vi "filtering_and_quant_demoinfocom.vi"(9 "Parity Size":dbl, 10 "Quantization rate":dbl) -> (0 "correlation coefficient r":dbl format="%.7g", 1 "SDR1 Key before ECC":u8[](array[numeric]), 2 "SDR2 Key before ECC":u8[](array[numeric]), 3 "CR rate":dbl[](array[numeric]), 4 "SDR2 Key After ECC":u8[](array[numeric]), 5 "Size of RS parity":u32, 6 "SDR1 Key after ECC":u8[](array[numeric]))   [LabVIEW 2021]
uses:
  system stop_demoinfocom.vi
  <vilib>/gmath/NI_Gmath.lvlib
panel:
  out "size after MQ":u32
  out "size after ECC":i32
  out "Size":dbl
  out "Filtered Signal":dbl[](array[numeric])
  out "output array size":u32
  in  "Python path":path=path "C:/Users/prashanth/Documents/GitHub/CR_Quantization/labview_demo_continuous.py"
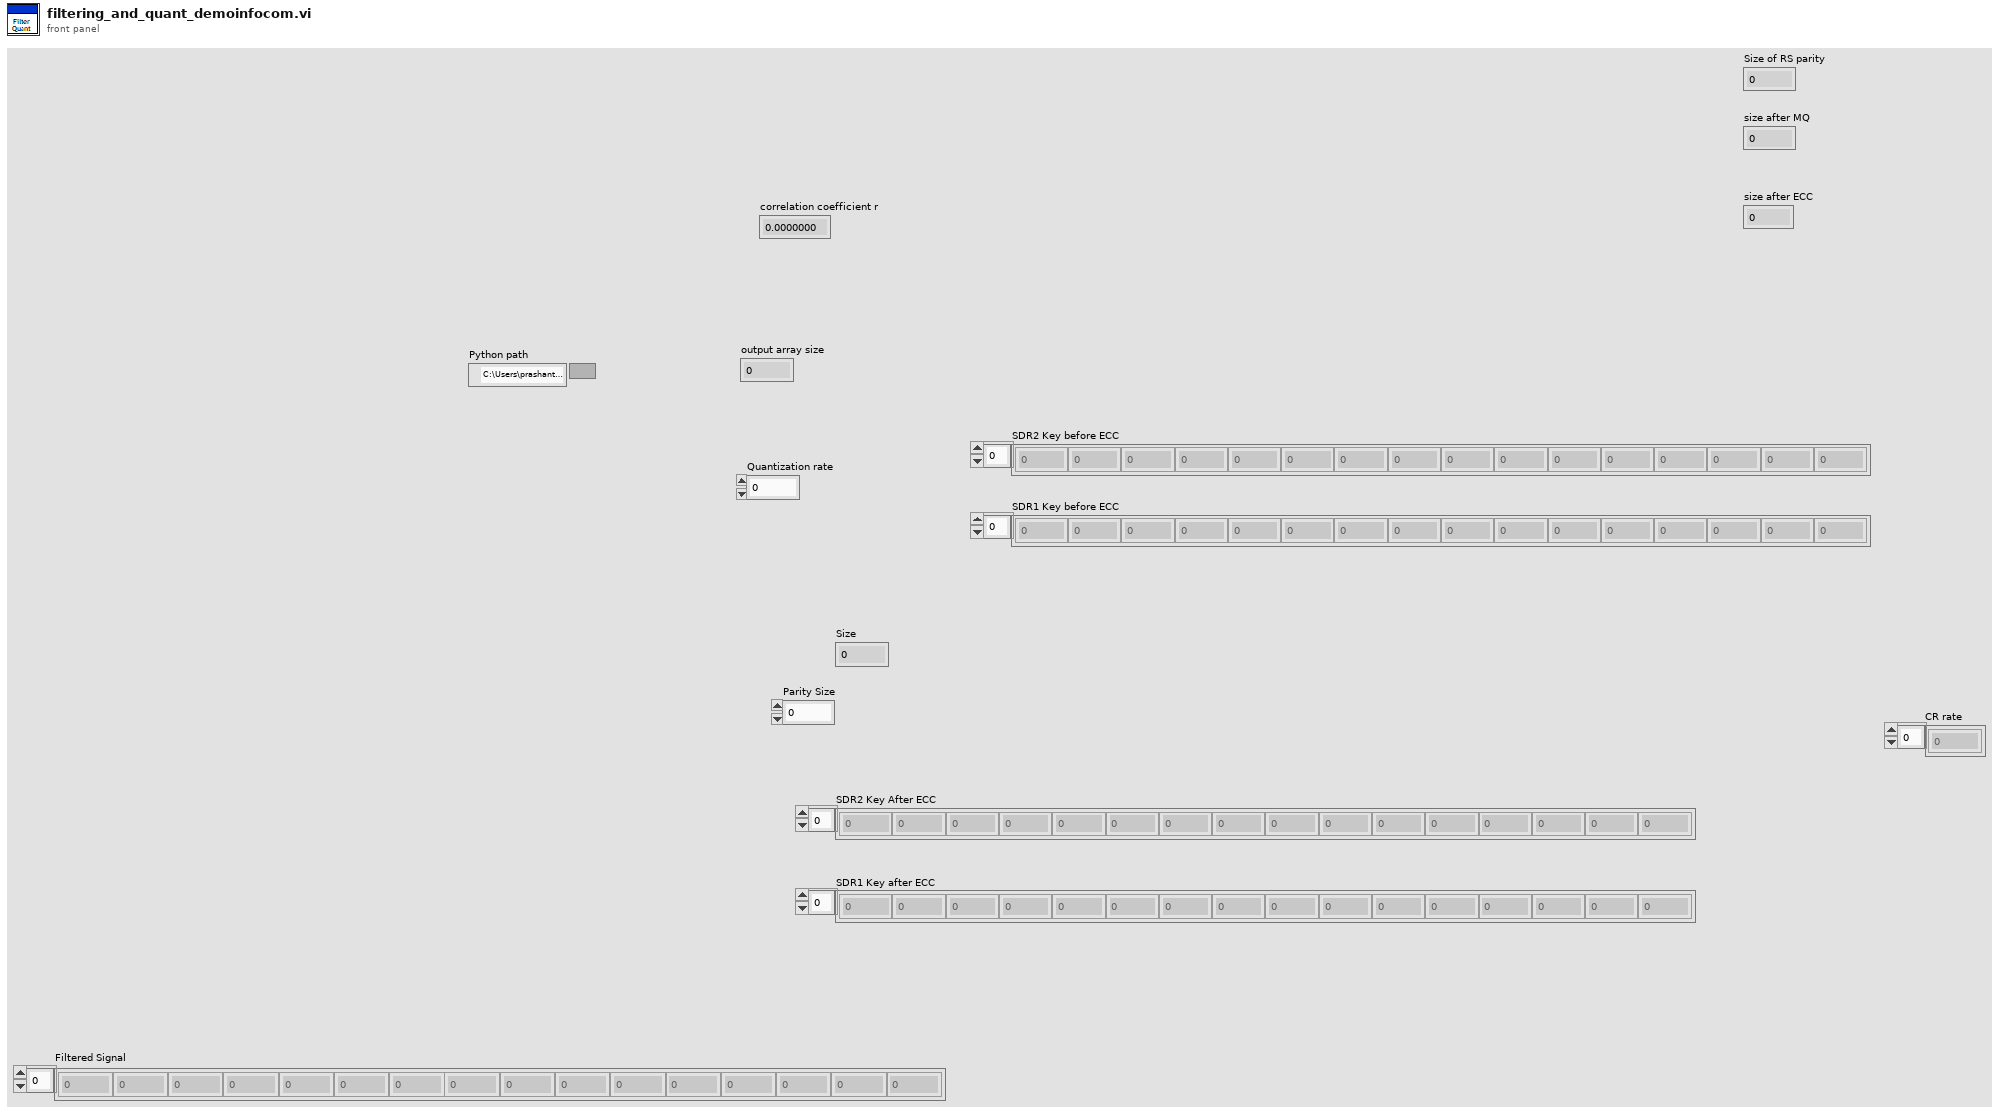
[diagram p1: front panel]
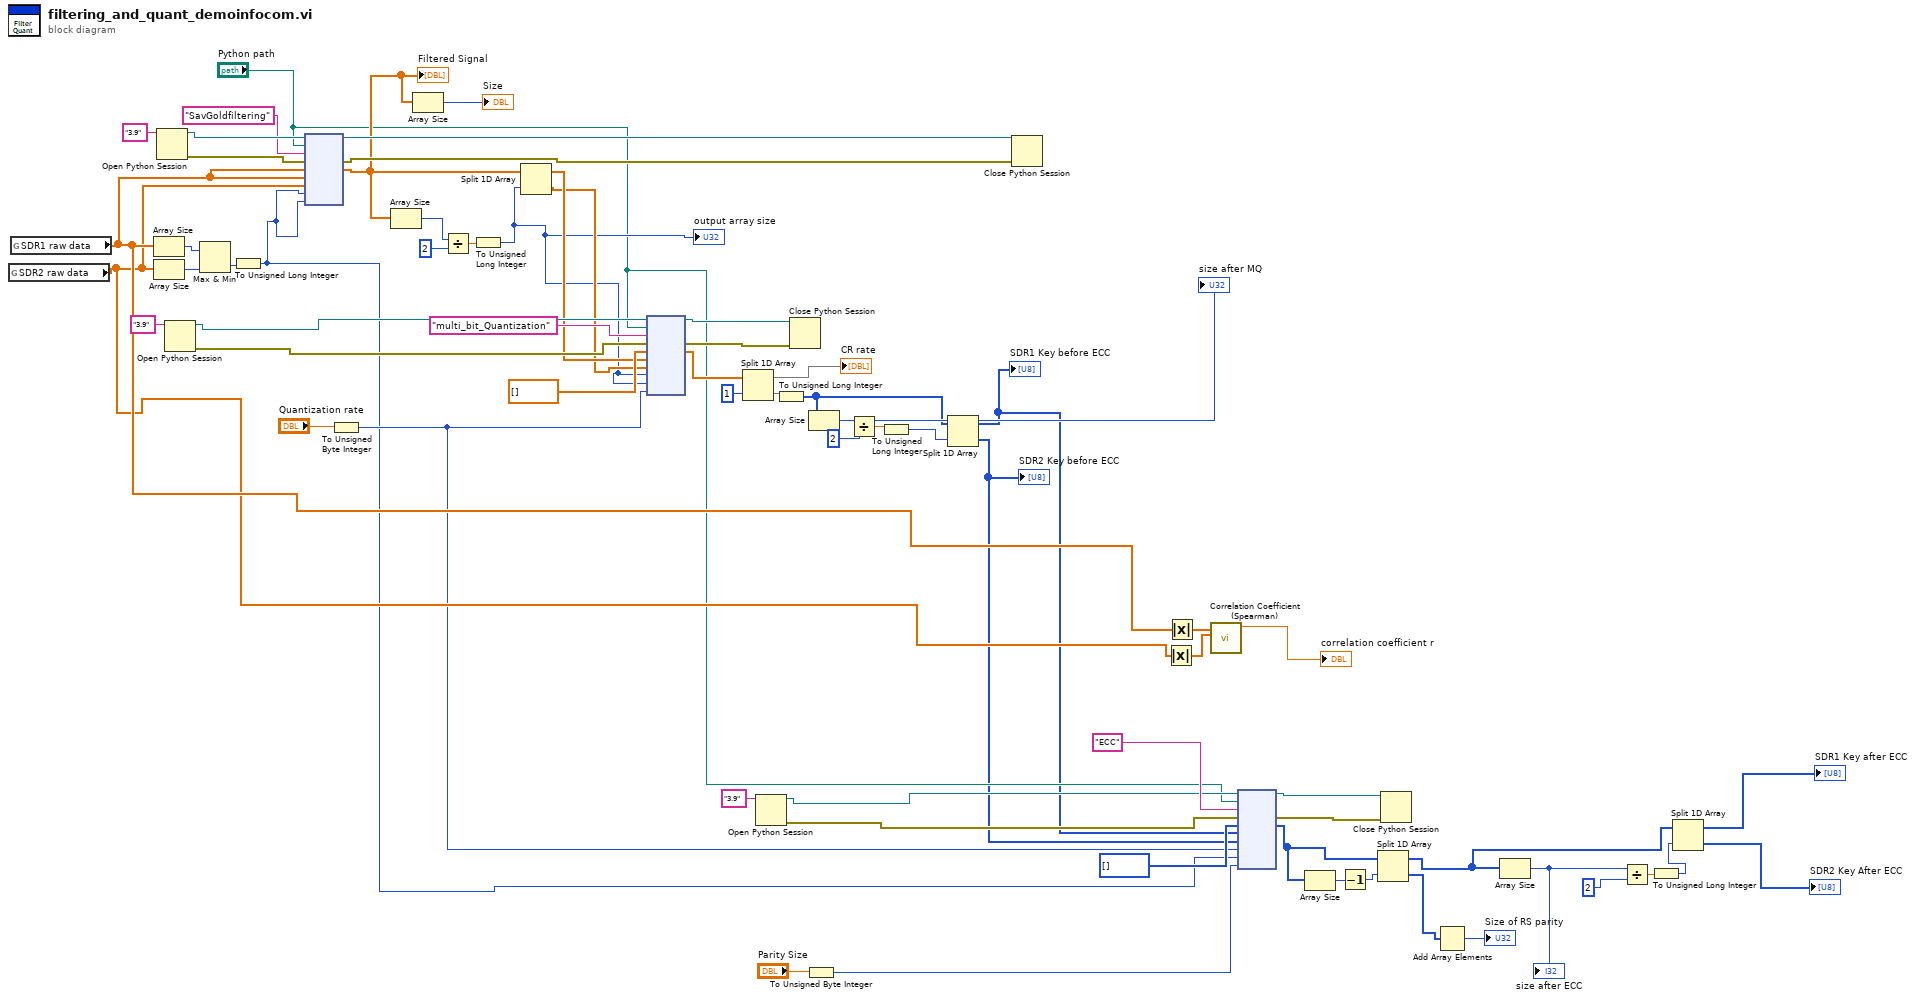
[diagram p0: block diagram]
diagram:
  n1 = global read "system stop_demoinfocom.vi" "SDR2 raw data"() -> (w30:dbl[])
  n2 = global read "system stop_demoinfocom.vi" "SDR1 raw data"() -> (w31:dbl[])
  n3 = Array Size(array=w31) -> (size(s)=w42:i32)
  n4 = Array Size(array=w30) -> (size(s)=w43:i32)
  n5 = Open Python Session(python version="3.9" ("Python version")) -> (session out=w65:refnum<k35>, error out=w63:errorcluster)  [unwired: 2 in]
  n6 = Open Python Session(python version="3.9" ("Python version")) -> (session out=w56:refnum<k35>, error out=w55:errorcluster)  [unwired: 2 in]
  n7 = Max & Min(x=w42, y=w43) -> (min(x,y)=w36:i32)  [unwired: 1 out]
  n8 = To Unsigned Long Integer(number=w36) -> (unsigned 32bit integer=w11:u32)
  n9 = node(w65, "Python path", "SavGoldfiltering" ("function name"), w63, w31, w31, w30, w11, w11) -> (w64:refnum<k35>, w50:errorcluster, w38:dbl[])  [unwired: 4 in, 2 out]
  "Filtered Signal" <- w38
  n10 = To Unsigned Byte Integer(number="Quantization rate") -> (unsigned 8bit integer=w12:u8)
  n11 = Array Size(array=w38) -> (size(s)=w51:i32)
  n12 = Array Size(array=w38) -> (size(s)=→"Size":i32)
  n13 = Divide(x=w51, y=2) -> (x/y=w59:dbl)
  n14 = To Unsigned Long Integer(number=w59) -> (unsigned 32bit integer=w41:u32)
  "output array size" <- w41
  n15 = Split 1D Array(array=w38, index=w41) -> (first subarray=w53:dbl[], second subarray=w52:dbl[])
  n16 = node(w56, "Python path", "multi_bit_Quantization" ("function name"), w55, dbl[] [], w53, w52, w41, w41, w12) -> (w49:refnum<k35>, w48:errorcluster, w46:dbl[])  [unwired: 5 in, 2 out]
  n17 = Split 1D Array(array=w46, index=1) -> (first subarray=→"CR rate":dbl[], second subarray=w33:dbl[])
  n18 = Open Python Session(python version="3.9" ("Python version")) -> (session out=w24:refnum<k35>, error out=w23:errorcluster)  [unwired: 2 in]
  n19 = To Unsigned Long Integer(number=w33) -> (unsigned 32bit integer=w32:u32[])
  n20 = Close Python Session(session in=w49, error in=w48) -> ()  [unwired: 1 out]
  n21 = To Unsigned Byte Integer(number="Parity Size") -> (unsigned 8bit integer=w10:u8)
  n22 = Array Size(array=w32) -> (size(s)=w45:i32)
  "size after MQ" <- w45
  n23 = Divide(x=w45, y=2) -> (x/y=w40:dbl)
  n24 = To Unsigned Long Integer(number=w40) -> (unsigned 32bit integer=w39:u32)
  n25 = Split 1D Array(array=w32, index=w39) -> (first subarray=w1:u32[], second subarray=w2:u32[])
  "SDR1 Key before ECC" <- w1
  "SDR2 Key before ECC" <- w2
  n26 = Close Python Session(session in=w64, error in=w50) -> ()  [unwired: 1 out]
  n27 = Absolute Value(x=w30) -> (abs(x)=w28:dbl[])
  n28 = Absolute Value(x=w31) -> (abs(x)=w29:dbl[])
  n29 = call <vilib>:"Correlation Coefficient (Spearman).vi"("Y"=w28, "X"=w29) -> ("correlation coefficient r"=→"correlation coefficient r":dbl)  [unwired: 8 in, 1 out]
  n30 = node(w24, "Python path", "ECC" ("function name"), w23, u32[] [], w1, w2, w12, w11, w10) -> (w21:refnum<k35>, w20:errorcluster, w8:u32[])  [unwired: 5 in, 2 out]
  n31 = Array Size(array=w8) -> (size(s)=w6:i32)
  n32 = Decrement(x=w6) -> (x-1=w5:i32)
  n33 = Split 1D Array(array=w8, index=w5) -> (first subarray=w7:u32[], second subarray=w4:u32[])
  n34 = Close Python Session(session in=w21, error in=w20) -> ()  [unwired: 1 out]
  n35 = Add Array Elements(numeric array=w4) -> (sum=→"Size of RS parity":u32)
  n36 = Array Size(array=w7) -> (size(s)=w9:i32)
  "size after ECC" <- w9
  n37 = Divide(x=w9, y=2) -> (x/y=w17:dbl)
  n38 = To Unsigned Long Integer(number=w17) -> (unsigned 32bit integer=w16:u32)
  n39 = Split 1D Array(array=w7, index=w16) -> (first subarray=→"SDR1 Key after ECC":u32[], second subarray=→"SDR2 Key After ECC":u32[])
